vi "Retention prune.vi"(8 "error in (no error)":errorcluster) -> (0 "error out":errorcluster)   [LabVIEW 2026, in "Tests.lvlib"]
doc: "Unit test (Caraya) for retention selection.\nVerifies that PruneSelection groups files by baseName, keeps the newest maxFileCount in each group, and returns the older surplus as FilesToDelete, so retention is oldest-first and per-series: files with different base names in one folder never prune against each other. Also verifies that maxFileCount = -1 keeps all.\nPure test: synthetic Path arrays, no file I/O, no fixture. Reaches the protected helper via the Tests.lvlib friend relationship.\n\nImplements LMBR-T-040, T-041 -> SRS-034. Assert-level IDs: Test-ID-Assert-Checklist.md."
uses:
  Tests.lvlib
  <vilib>/addons/_JKI Toolkits/Caraya/classes/Assert/Assert Equal Value_Variant.vi
  <vilib>/addons/_JKI Toolkits/Caraya/classes/Assert/Assert False.vi
  <vilib>/addons/_JKI Toolkits/Caraya/classes/Test/Test.lvclass
  src/Lumberjack.lvlib
  <vilib>/addons/_JKI Toolkits/Caraya/classes/Assert/Assert.lvclass
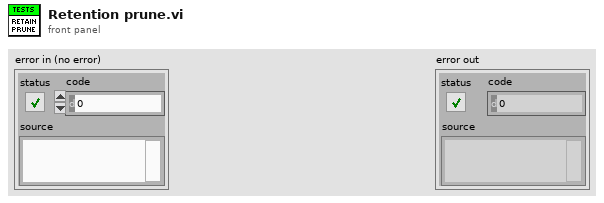
[diagram p1: front panel]
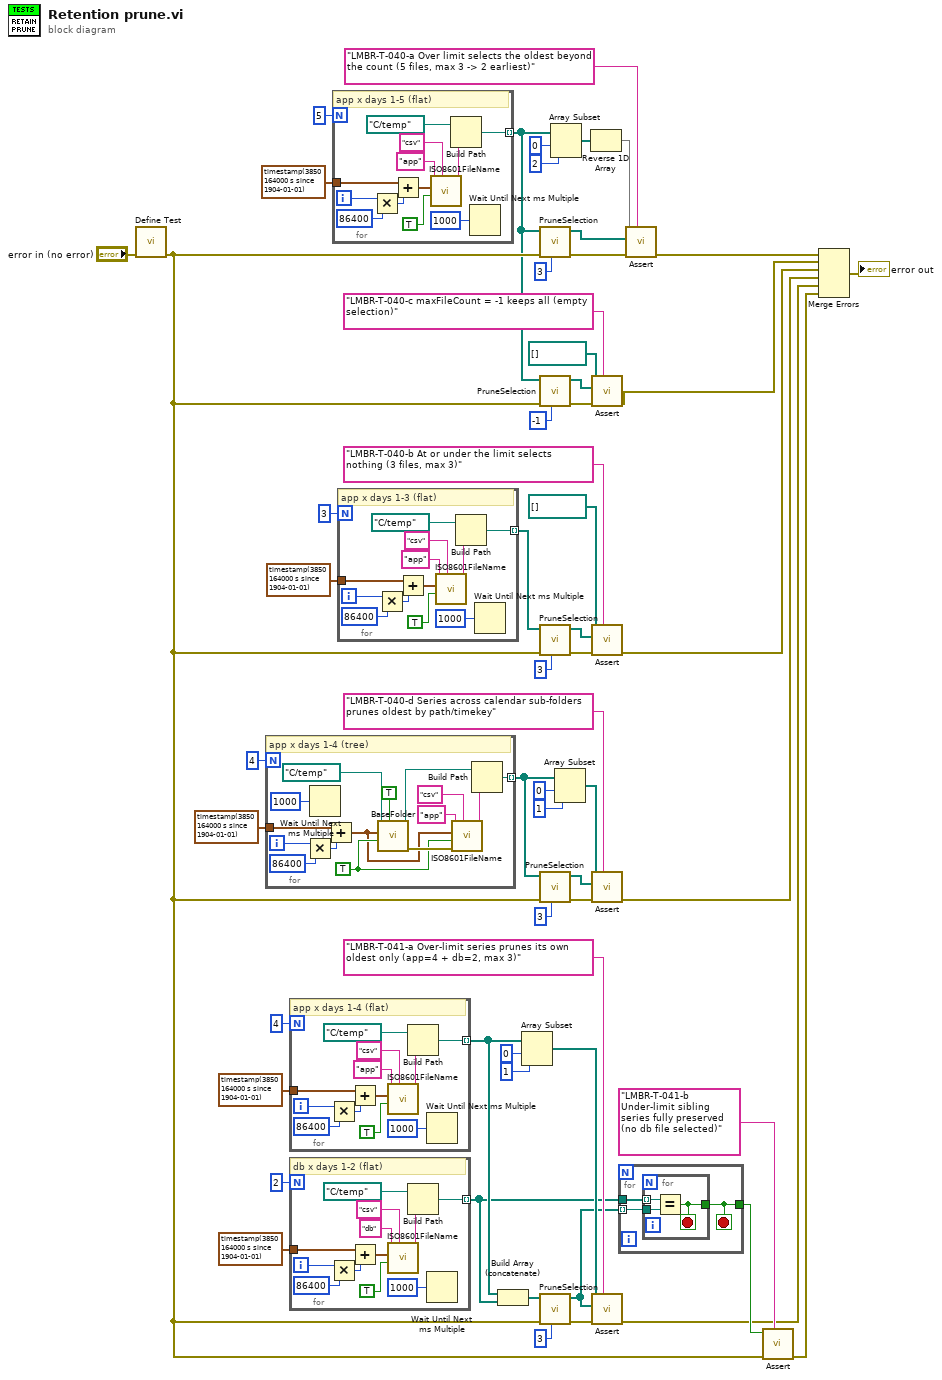
[diagram p0: block diagram]
diagram:
  n1 = call <vilib>:"Define Test.vi"("error in (no error)"="error in (no error)") -> ("error out"=w37:errorcluster)  [unwired: 9 in, 1 out]
  n2 = for {
    N: 4 -> [_]
    tunnel: timestamp(3850164000 s since 1904-01-01) -> [w71]
    tunnel: [w60] -> w3 mode=indexing
    i -> [w73]
    w62 = TRUE ("useUTC")
    # "app x days 1-4 (tree)"
    n3 = Multiply(x=w73, y=86400) -> (x*y=w70:i32)
    n4 = Wait Until Next ms Multiple(millisecond multiple=u32 1000) -> ()  [unwired: 1 out]
    n5 = Add(x=w71, y=w70) -> (x+y=w61:timestamp)
    n6 = call "BaseFolder.vi"("calendarFolderTree"=TRUE, "useUTC"=w62, "Timestamp"=w61, "RootFolder"=path "C:/temp") -> ("error out"=w63:errorcluster, "Folder"=w66:path)  [unwired: 6 in]
    n7 = call "ISO8601FileName.vi"("Extension"="csv", "error in (no error)"=w63, "useUTC"=w62, "Timestamp"=w61, "BaseName"="app") -> ("FileName"=w65:string)  [unwired: 5 in, 1 out]
    n8 = Build Path(base path=w66, name or relative path=w65) -> (appended path=w60:path)
  }
  n9 = for {
    N: 4 -> [_]
    tunnel: timestamp(3850164000 s since 1904-01-01) -> [w83]
    tunnel: [w76] -> w52 mode=indexing
    i -> [w85]
    # "app x days 1-4 (flat)"
    n10 = Multiply(x=w85, y=86400) -> (x*y=w82:i32)
    n11 = Add(x=w83, y=w82) -> (x+y=w77:timestamp)
    n12 = call "ISO8601FileName.vi"("Extension"="csv", "useUTC"=TRUE, "Timestamp"=w77, "BaseName"="app") -> ("FileName"=w79:string)  [unwired: 6 in, 1 out]
    n13 = Build Path(base path=path "C:/temp" ("RootFolder"), name or relative path=w79) -> (appended path=w76:path)
    n14 = Wait Until Next ms Multiple(millisecond multiple=u32 1000) -> ()  [unwired: 1 out]
  }
  n15 = for {
    N: 2 -> [_]
    tunnel: timestamp(3850164000 s since 1904-01-01) -> [w95]
    tunnel: [w88] -> w38 mode=indexing
    i -> [w97]
    # "db x days 1-2 (flat)"
    n16 = Multiply(x=w97, y=86400) -> (x*y=w94:i32)
    n17 = Add(x=w95, y=w94) -> (x+y=w89:timestamp)
    n18 = call "ISO8601FileName.vi"("Extension"="csv", "useUTC"=TRUE, "Timestamp"=w89, "BaseName"="db") -> ("FileName"=w91:string)  [unwired: 6 in, 1 out]
    n19 = Build Path(base path=path "C:/temp" ("RootFolder"), name or relative path=w91) -> (appended path=w88:path)
    n20 = Wait Until Next ms Multiple(millisecond multiple=u32 1000) -> ()  [unwired: 1 out]
  }
  n21 = for {
    N: 5 -> [_]
    tunnel: timestamp(3850164000 s since 1904-01-01) -> [w107]
    tunnel: [w100] -> w9 mode=indexing
    i -> [w109]
    # "app x days 1-5 (flat)"
    n22 = Multiply(x=w109, y=86400) -> (x*y=w106:i32)
    n23 = Add(x=w107, y=w106) -> (x+y=w101:timestamp)
    n24 = call "ISO8601FileName.vi"("Extension"="csv", "useUTC"=TRUE, "Timestamp"=w101, "BaseName"="app") -> ("FileName"=w103:string)  [unwired: 6 in, 1 out]
    n25 = Build Path(base path=path "C:/temp" ("RootFolder"), name or relative path=w103) -> (appended path=w100:path)
    n26 = Wait Until Next ms Multiple(millisecond multiple=u32 1000) -> ()  [unwired: 1 out]
  }
  n27 = for {
    N: 3 -> [_]
    tunnel: timestamp(3850164000 s since 1904-01-01) -> [w119]
    tunnel: [w112] -> w16 mode=indexing
    i -> [w121]
    # "app x days 1-3 (flat)"
    n28 = Multiply(x=w121, y=86400) -> (x*y=w118:i32)
    n29 = Add(x=w119, y=w118) -> (x+y=w113:timestamp)
    n30 = call "ISO8601FileName.vi"("Extension"="csv", "useUTC"=TRUE, "Timestamp"=w113, "BaseName"="app") -> ("FileName"=w115:string)  [unwired: 6 in, 1 out]
    n31 = Build Path(base path=path "C:/temp" ("RootFolder"), name or relative path=w115) -> (appended path=w112:path)
    n32 = Wait Until Next ms Multiple(millisecond multiple=u32 1000) -> ()  [unwired: 1 out]
  }
  n33 = Build Array (concatenate)(w52, w38) -> (w40:path[])
  n34 = Array Subset(array=w52, index=0, length=1) -> (w48:path[])
  n35 = call "PruneSelection.vi"("maxFileCount"=3, "error in (no error)"=w37, "ExistingFiles"=w9) -> ("error out"=w25:errorcluster, "FilesToDelete"=w24:path[])  [unwired: 7 in]
  n36 = call "PruneSelection.vi"("maxFileCount"=-1, "error in (no error)"=w37, "ExistingFiles"=w9) -> ("error out"=w13:errorcluster, "FilesToDelete"=w12:path[])  [unwired: 7 in]
  n37 = call "PruneSelection.vi"("maxFileCount"=3, "error in (no error)"=w37, "ExistingFiles"=w16) -> ("error out"=w21:errorcluster, "FilesToDelete"=w20:path[])  [unwired: 7 in]
  n38 = call "PruneSelection.vi"("maxFileCount"=3, "error in (no error)"=w37, "ExistingFiles"=w3) -> ("error out"=w7:errorcluster, "FilesToDelete"=w6:path[])  [unwired: 7 in]
  n39 = call "PruneSelection.vi"("maxFileCount"=3, "error in (no error)"=w37, "ExistingFiles"=w40) -> ("error out"=w50:errorcluster, "FilesToDelete"=w39:path[])  [unwired: 7 in]
  n40 = Array Subset(array=w9, index=0, length=2) -> (w2:path[])
  n41 = Array Subset(array=w3, index=0, length=1) -> (w4:path[])
  n42 = Reverse 1D Array(array=w2) -> (reversed array=w1:path[])
  n43 = call-poly <vilib>:"Assert.vi"("Label"="LMBR-T-040-c maxFileCount = -1 keeps all (empty selection)", "error in (no error)"=w13, "Actual"=w12, "Expected"=path[] []) -> ("error out"=w46:errorcluster)  [unwired: 6 in, 1 out]
  n44 = call-poly <vilib>:"Assert.vi"("Label"="LMBR-T-040-b At or under the limit selects nothing (3 files, max 3)", "error in (no error)"=w21, "Actual"=w20, "Expected"=path[] []) -> ("error out"=w44:errorcluster)  [unwired: 6 in, 1 out]
  n45 = call-poly <vilib>:"Assert.vi"("Label"="LMBR-T-040-d Series across calendar sub-folders prunes oldest by path/timekey", "error in (no error)"=w7, "Actual"=w6, "Expected"=w4) -> ("error out"=w43:errorcluster)  [unwired: 6 in, 1 out]
  n46 = call-poly <vilib>:"Assert.vi"("Label"="LMBR-T-041-a Over-limit series prunes its own oldest only (app=4 + db=2, max 3)", "error in (no error)"=w50, "Actual"=w39, "Expected"=w48) -> ("error out"=w35:errorcluster)  [unwired: 6 in, 1 out]
  n47 = for {
    tunnel: w38 -> [w124]
    tunnel: w39 -> [w125] mode=indexing
    tunnel: [w123] -> w42
    stop <- w123 stop-if-true
    n48 = for {
      tunnel: w125 -> [w128]
      tunnel: w124 -> [w127] mode=indexing
      tunnel: [w126] -> w123
      stop <- w126 stop-if-true
      n49 = Equal?(x=w127, y=w128) -> (x = y?=w126:bool)
    }
  }
  n50 = call-poly <vilib>:"Assert.vi"("Label"="LMBR-T-040-a Over limit selects the oldest beyond the count (5 files, max 3 -> 2 earliest)", "error in (no error)"=w25, "Actual"=w24, "Expected"=w1) -> ("error out"=w47:errorcluster)  [unwired: 6 in, 1 out]
  n51 = call-poly <vilib>:"Assert.vi"("Label"="LMBR-T-041-b Under-limit sibling series fully preserved (no db file selected)", "error in (no error)"=w37, "False?"=w42) -> ("error out"=w36:errorcluster)  [unwired: 7 in, 1 out]
  n52 = Merge Errors(w47, w46, w44, w43, w35, w36) -> (→"error out":errorcluster)
